vi "Connect.vi"(6 "error in":errorcluster, 7 "Address":string, 9 "Websocket Handler in":refnum<class "Websocket Handler.lvclass">) -> (0 "error out":errorcluster, 3 "Websocket Handler out":refnum<class "Websocket Handler.lvclass">)   [LabVIEW 2020, in "wamplv.lvlib" / "Websocket Handler.lvclass"]
uses:
  Websocket Handler.lvclass
  C:/local/wamplv/CommHandlerBase/CommHandlerBase.lvclass
  <vilib>/MediaMongrels Ltd/WebSockets/WebSockets/WebSocket/WebSocket.lvclass/WebSocket.ctl
  Websocket Handler.lvclass/Websocket Handler.ctl
  <vilib>/MediaMongrels Ltd/WebSockets/WebSockets/WebSocket/Write Protocols.vi
  <vilib>/MediaMongrels Ltd/WebSockets/WebSockets/WebSocket Client/WebSocket Client.lvclass
  C:/Program Files (x86)/National Instruments/LabVIEW 2020/vi.lib/MediaMongrels Ltd/WebSockets/WebSockets/WebSocket/WebSocket.lvclass
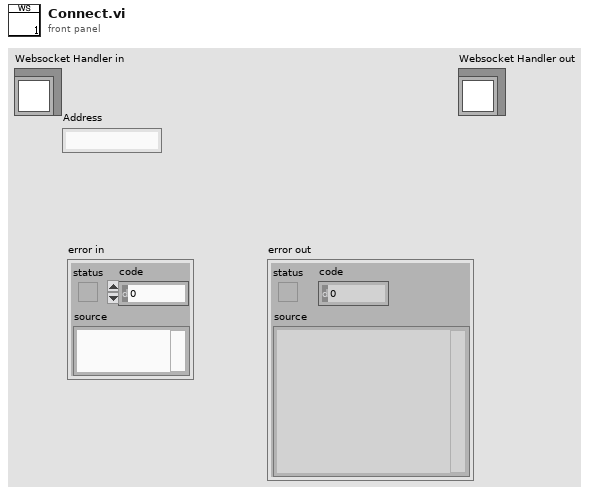
[diagram p1: front panel]
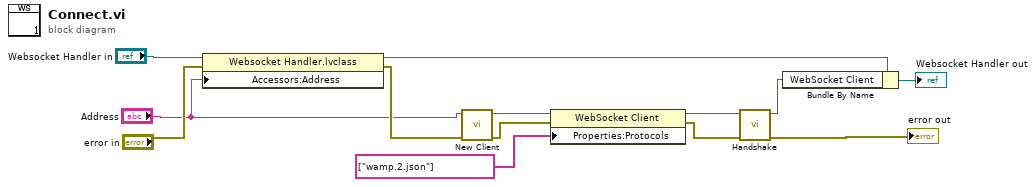
[diagram p0: block diagram]
diagram:
  n1 = property class="Websocket Handler.lvclass"(reference="Websocket Handler in", error in="error in", "Accessors:Address"="Address") -> (reference out=w2:refnum<class "Websocket Handler.lvclass">, error out=w3:errorcluster)
  n2 = call <vilib>:"New Client.vi"("error in (no error)"=w3, "WebSocket URL"="Address") -> ("error out"=w7:errorcluster, "WebSocket Client out"=w10:refnum<class "WebSocket Client.lvclass">)  [unwired: 8 in]
  n3 = property class="WebSocket Client"(reference=w10, error in=w7, "Properties:Protocols"=string[] ["wamp.2.json"] ("Protocols")) -> (reference out=w9:refnum<class "WebSocket Client.lvclass">, error out=w6:errorcluster)
  n4 = call-dynamic "Handshake.vi"("error in (no error)"=w6, "WebSocket Client in"=w9) -> ("error out"=→"error out":errorcluster, "WebSocket Client out"=w11:refnum<class "WebSocket Client.lvclass">)  [unwired: 8 in]
  n5 = Bundle By Name(cluster=w2, "WebSocket Client"=w11) -> (→"Websocket Handler out":refnum<class "Websocket Handler.lvclass">)
